vi "Volt Reader Trigger9.vi"() -> ()   [LabVIEW 2014]
uses:
  Enum State Machine Typedef.ctl
  <vilib>/Utility/error.llb/DialogType.ctl
  <vilib>/_DAQmxBase/Internals/DAQmxBase Create Channel (AI-Voltage-Basic).vi
  <vilib>/_DAQmxBase/Internals/DAQmxBase Timing (Sample Clock).vi
  <vilib>/measure/mamon.llb/Trigger Detection for 1 Channel.vi
  <vilib>/_DAQmxBase/Internals/DAQmxBase Read (Analog 2D DBL NChan NSamp).vi
  <vilib>/measure/NI_MAPro.lvlib
panel:
  out "trigger location":dbl
  in  "Timeout (in iterations)":i16
  out "State":T1
  out "Raw Waveform":waveform(dbl)(graph)
  out "Waveform Graph":waveform(dbl)(graph)
  in  "Buffer (Seconds)":dbl
  out "Threshold":dbl
  in  "units":i32(ring)=10348 items=["Volts"=10348, "From Custom Scale"=10065]
  in  "stop":bool
  in  "physical channels":tag
  in  "maximum value":dbl=5.0 format="%0.2f"
  in  "minimum value":dbl=-5.0 format="%0.2f"
  in  "rate":i32=1000 caption="Sample Rate"
  # "The inputs above MUST BE\nPreset before running"
  # "NOTE: Just change the Y axis value"
  # "Make Sure that Buffer does not equal 0"
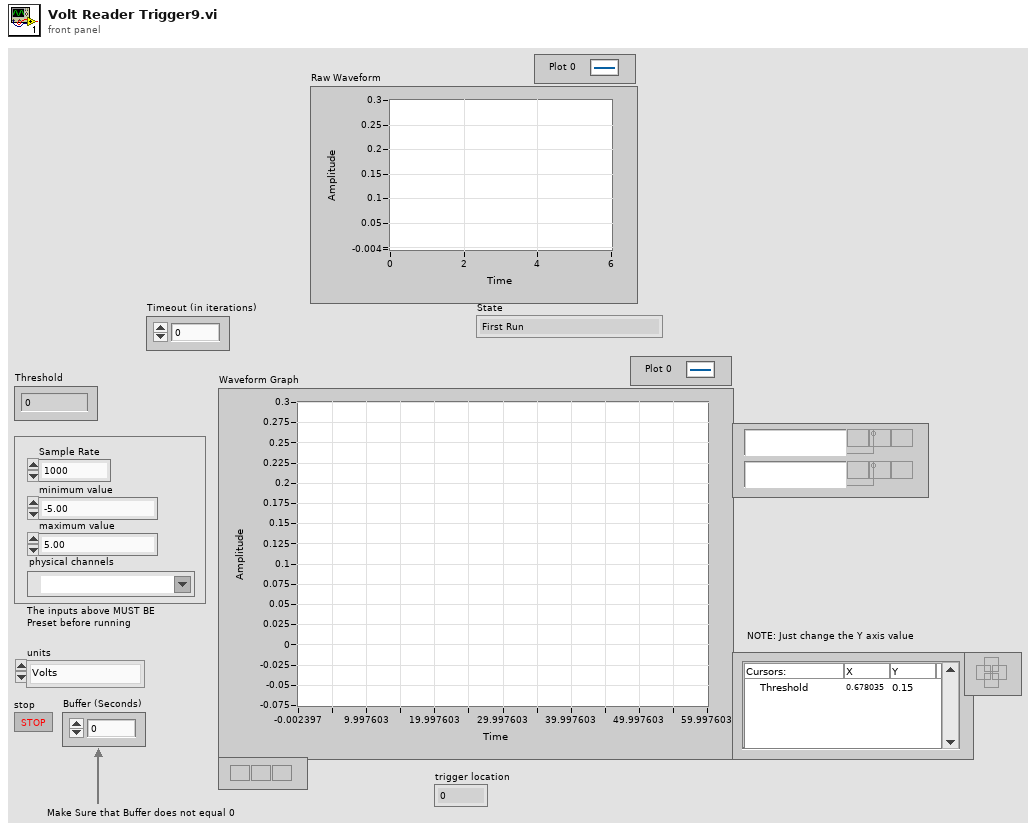
[diagram p1: front panel]
types:
  T1 = typedef "Enum State Machine Typedef.ctl" = enum16{"First Run", "Gather and Edit Data", "Find Max with Gather Data", "Trigger Occured", "Found the Max", "Just Displayed", "The Max is in the Middle", "Base State", "Timeout"}
  T2 = typedef "DialogType.ctl" = u16
  T3 = typedef "LVCursorListTypeDef.ctl" = cluster{"Name":string, "Color":u32, "Style":u8, "Point Style":u8, "Name Visible":bool, "Allow Drag":bool, "Cursor Mode":u32, "Plot":i32, "Index":i32, "Position":cluster{"X":dbl, "Y":dbl}, "X Scale":u32, "Y Scale":u32, "Watch Plots":i32[], "Watch All Plots":bool, "Plot Area":i32, "Label Offset":cluster{"X":dbl, "Y":dbl}}[]
  T4 = cluster{"Name":string, "Color":u32, "Style":u8, "Point Style":u8, "Name Visible":bool, "Allow Drag":bool, "Cursor Mode":u32, "Plot":i32, "Index":i32, "Position":cluster{"X":dbl, "Y":dbl}, "X Scale":u32, "Y Scale":u32, "Watch Plots":i32[], "Watch All Plots":bool, "Plot Area":i32, "Label Offset":cluster{"X":dbl, "Y":dbl}}
  T5 = enum16{"In the Center Range", "Before the Center Range", "After the Center Range"}
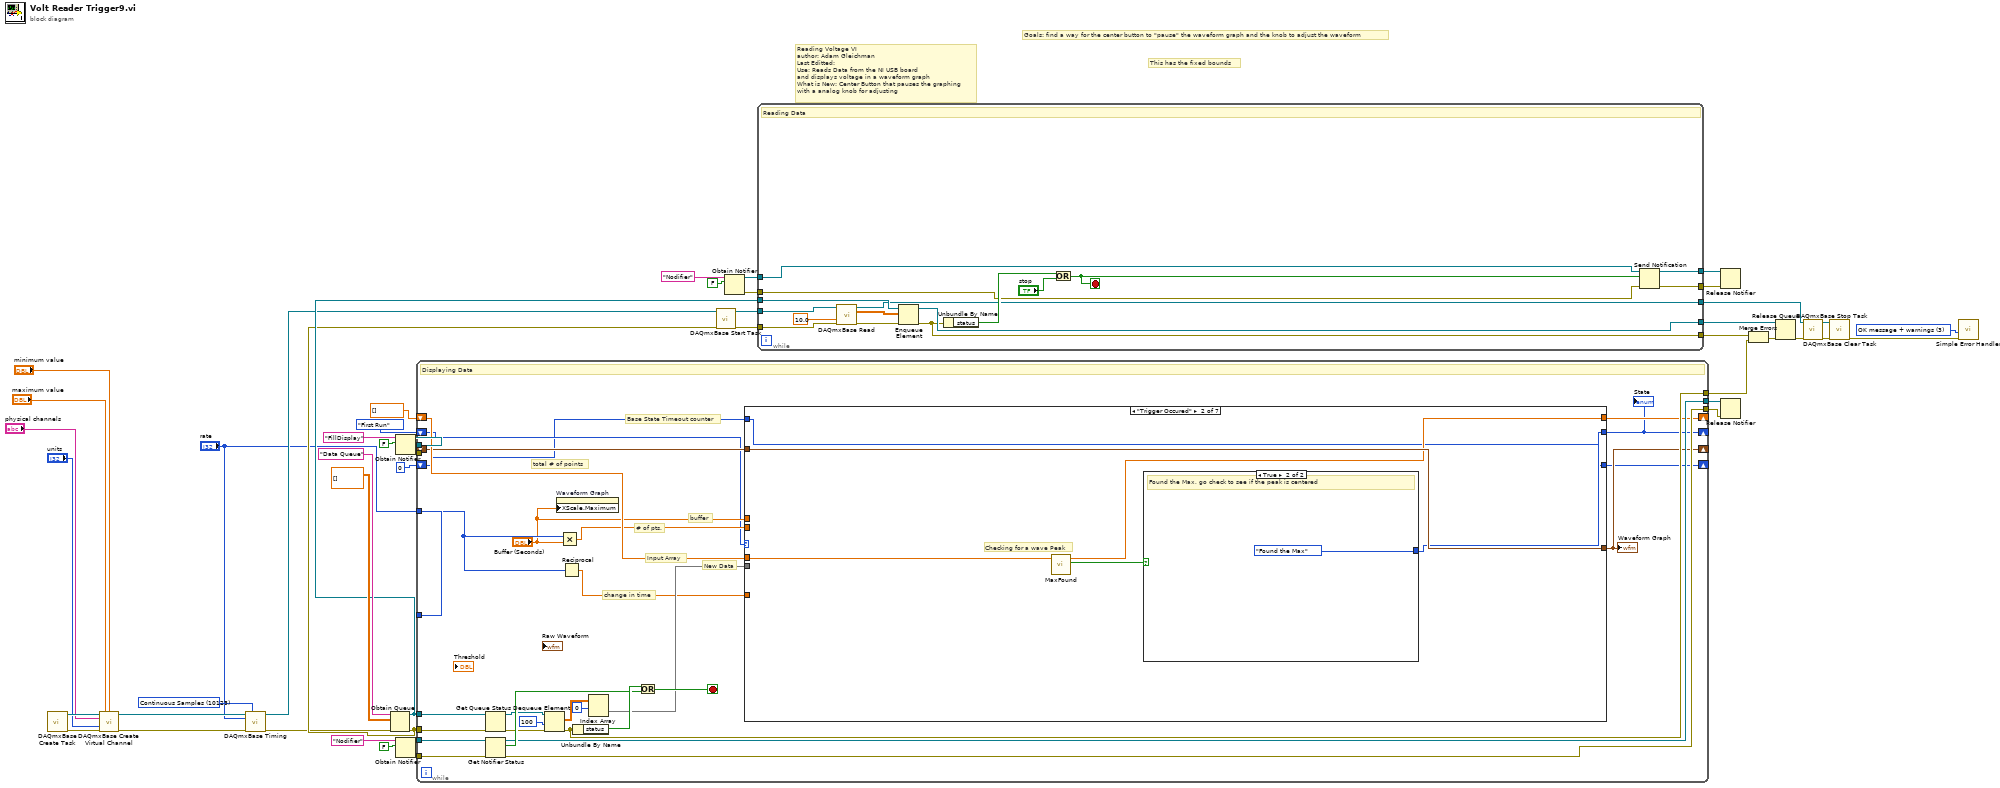
[diagram p0: block diagram]
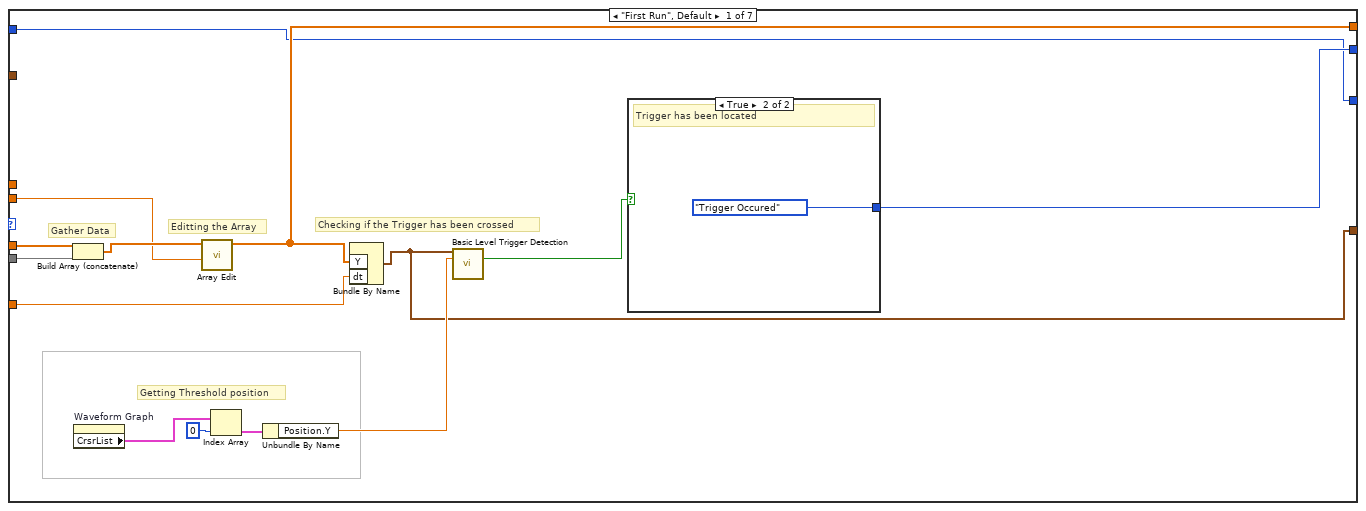
[diagram p2: hidden frame]
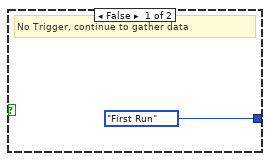
[diagram p3: hidden frame]
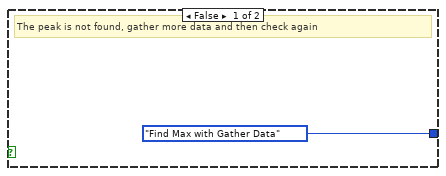
[diagram p4: hidden frame]
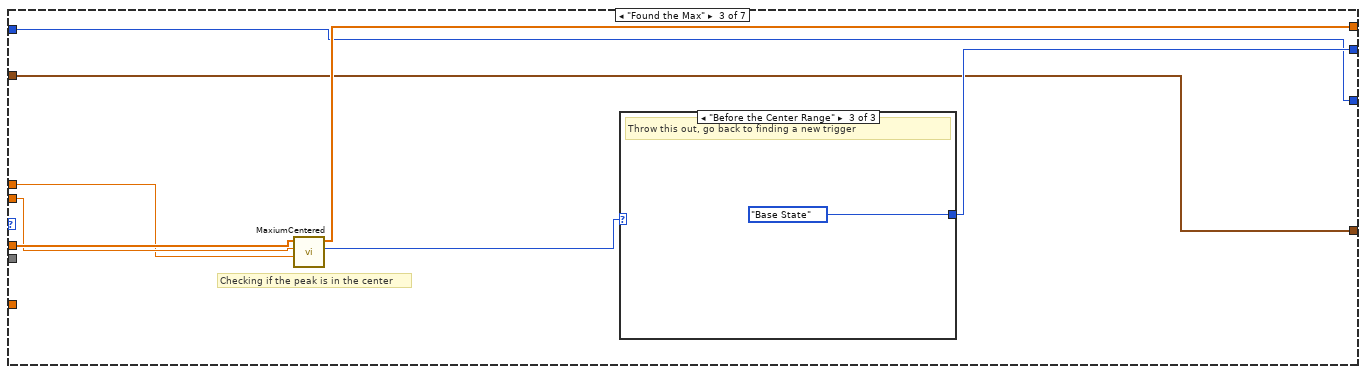
[diagram p5: hidden frame]
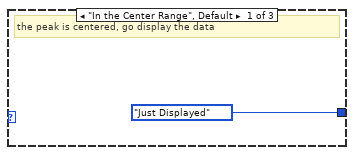
[diagram p6: hidden frame]
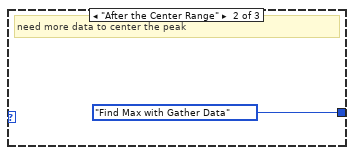
[diagram p7: hidden frame]
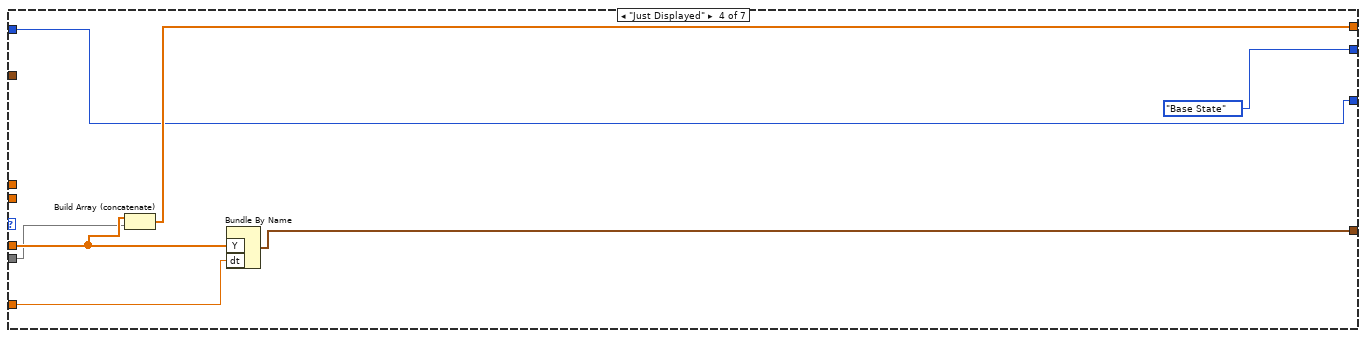
[diagram p8: hidden frame]
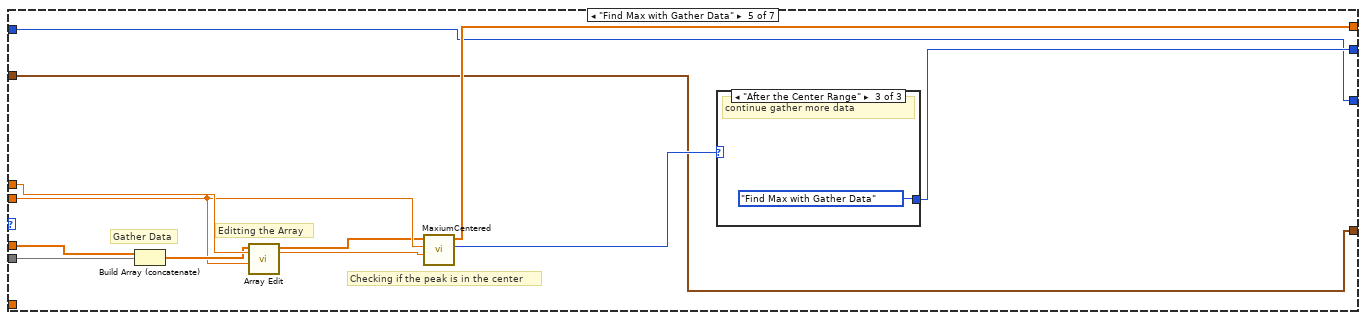
[diagram p9: hidden frame]
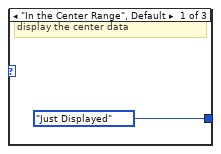
[diagram p10: hidden frame]
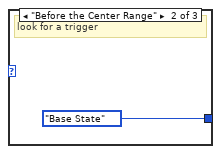
[diagram p11: hidden frame]
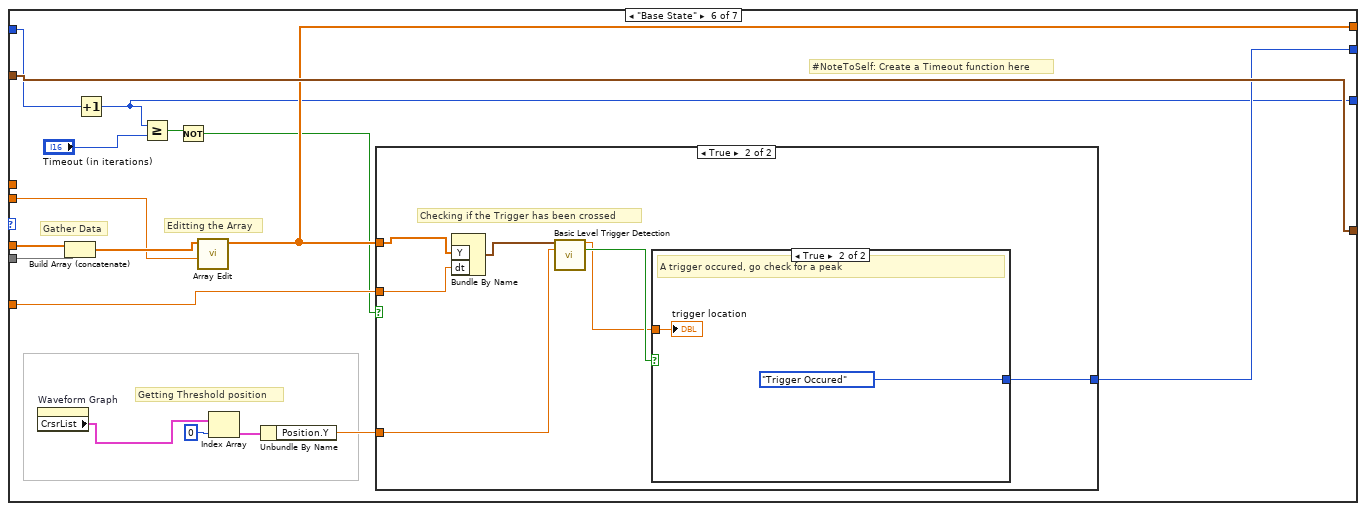
[diagram p12: hidden frame]
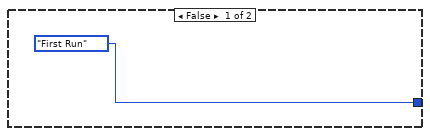
[diagram p13: hidden frame]
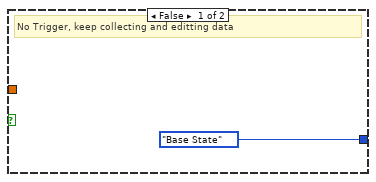
[diagram p14: hidden frame]
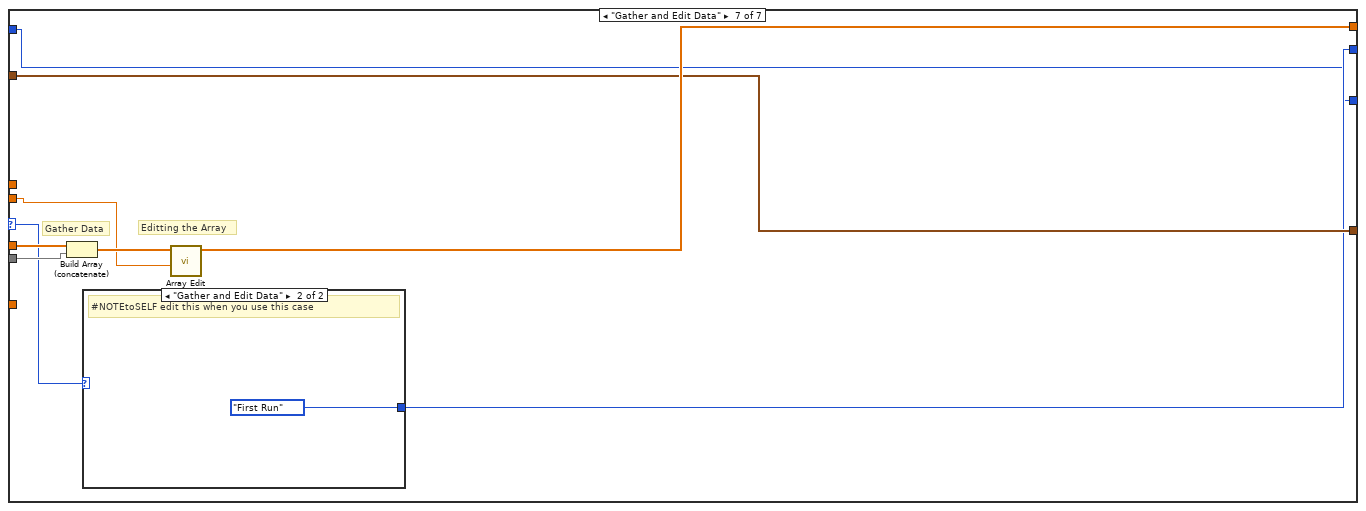
[diagram p15: hidden frame]
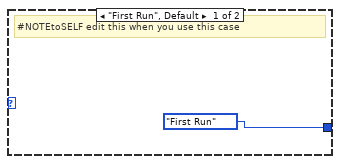
[diagram p16: hidden frame]
diagram:
  w24 = 10123 items=["Finite Samples"=10178, "Continuous Samples"=10123, "Hardware Timed Single Point"=12522] ("sample mode")
  w26 = T2 3 items=["no dialog", "OK message", "continue or stop message", "OK message + warnings", "continue/stop + warnings"] ("type of dialog (OK msg:1)")
  # "Goals: find a way for the center button to \"pause\" the waveform graph and the knob to adjust the waveform"
  # "This has the fixed bounds"
  # "Reading Voltage VI\nauthor: Adam Gleichman\nLast Editted: \nUse: Reads Data from the NI USB board\nand displays voltage in a waveform graph\nWhat is New: Center Button that pauses the graphing\nwith a analog knob for adjusting"
  n1 = call <vilib>:"DAQmxBase Create Task.vi"() -> ("task out"=w46:refnum<k21>, "error out"=w45:errorcluster)  [unwired: 5 in, 9 out]
  n2 = call-poly <vilib>:"DAQmxBase Create Virtual Channel.vi"("task in"=w46, "maximum value"="maximum value", "minimum value"="minimum value", "physical channels"="physical channels", "units"="units", "error in"=w45) -> ("task out"=w43:refnum<k21>, "error out"=w44:errorcluster)  [unwired: 3 in, 5 out]
  n3 = call-poly <vilib>:"DAQmxBase Timing.vi"("task/channels in"=w43, "sample mode"=w24, "rate"="rate", "error in"=w44) -> ("task out"=w12:refnum<k21>, "error out"=w11:errorcluster)  [unwired: 3 in, 7 out]
  n4 = Obtain Queue(name (unnamed)="Data Queue", element data type=dbl[][] [] ("data"), error in (no error)=w11) -> (queue out=w33:refnum<queue>, error out=w32:errorcluster)  [unwired: 2 in, 1 out]
  n5 = Obtain Notifier(name (unnamed)="FillDisplay", notification data type=FALSE) -> (notifier out=w8:refnum<notifier>, error out=w7:errorcluster)  [unwired: 2 in, 1 out]
  n6 = Obtain Notifier(name (unnamed)="Nodifier", notification data type=FALSE) -> (notifier out=w17:refnum<notifier>, error out=w15:errorcluster)  [unwired: 2 in, 1 out]
  n7 = while {
    tunnel: w33 -> [w75]
    tunnel: w32 -> [w64]
    tunnel: [w73] -> w31
    tunnel: w17 -> [w70]
    tunnel: w15 -> [w69]
    tunnel: [w67] -> w13
    tunnel: [w66] -> w14
    tunnel: "rate" -> [_]
    tunnel: "rate" -> [w60]
    shift-right: [w51] -> _
    shift-left: dbl[] [] -> [w59]
    tunnel: w8 -> [_]
    tunnel: w7 -> [_]
    shift-right: [w50] -> _
    shift-left: Enum_State_Machine_Typedef."First Run" -> [w53]
    shift-right: [w52] -> _
    shift-left: _ -> [w55]
    shift-right: [w48] -> _
    shift-left: 0 -> [w49]
    stop <- w71 stop-if-true
    # "Base State Timeout counter"
    # "change in time"
    # "buffer"
    # "New Data"
    # "Input Array"
    # "# of pts."
    # "total # of points"
    # "Displaying Data"
    n8 = Get Queue Status(queue=w75, error in (no error)=w64) -> (queue out=w65:refnum<queue>, error out=w63:errorcluster)  [unwired: 1 in, 6 out]
    n9 = Get Notifier Status(notifier=w70, error in (no error)=w69) -> (notifier out=w67:refnum<notifier>, current notification=w68:bool, error out=w66:errorcluster)  [unwired: 2 out]
    n10 = Dequeue Element(queue=w65, timeout in ms (-1)=100, error in (no error)=w63) -> (element=w61:dbl[][], error out=w73:errorcluster)  [unwired: 2 out]
    n11 = property on="Waveform Graph" class="WFGraph (strict)"("XScale.Maximum"="Buffer (Seconds)") -> ()  [unwired: 2 in, 2 out]
    n12 = Multiply(x=w60, y="Buffer (Seconds)") -> (x*y=w56:dbl)
    n13 = Reciprocal(x=w60) -> (1/x=w57:dbl)
    n14 = Unbundle By Name(w73) -> ("status"=w72:bool)
    n15 = Index Array(array=w61, index (row)=0 ("index")) -> (element=w58:dbl[])  [unwired: 1 in]
    n16 = Or(x=w72, y=w68) -> (x .or. y?=w71:bool)
    n17 = case shown="\"Trigger Occured\"" w53 {
      selector: w53 -> [_ _ _ _ _ _ w164]
      tunnel: w59 -> [w89 w97 w107 w116 w128 w148 w168]
      tunnel: w58 -> [w88 _ _ w115 w127 w147 w167]
      tunnel: w57 -> [w82 _ _ w117 _ w141 _]
      tunnel: w56 -> [w86 _ w106 _ w124 w145 w165]
      tunnel: [w79 w96 w101 w113 w119 w140 w162] -> w52
      tunnel: w55 -> [_ w96 w101 _ w119 w140 w162]
      tunnel: "Buffer (Seconds)" -> [_ _ w105 _ w126 _ _]
      tunnel: [w78 w94 w104 w114 w121 w138 w163] -> w51
      tunnel: [w77 w93 w102 Enum_State_Machine_Typedef."Base State" w120 w139 w161] -> w50
      tunnel: w49 -> [w76 w92 w100 w111 w118 w136 w160]
      tunnel: [w76 w92 w100 w111 w118 w132 w160] -> w48
      frame "First Run", Default {
        # "Checking if the Trigger has been crossed"
        # "Getting Threshold position"
        # "Editting the Array"
        # "Gather Data"
        n18 = Build Array (concatenate)(w89, w88) -> (w87:dbl[])
        n19 = property on="Waveform Graph" class="WFGraph (strict)"() -> ("CrsrList"=w84:T3)  [unwired: 2 in, 2 out]
        n20 = call "Array Edit.vi"("Number of Points"=w86, "Y-values"=w87) -> ("Editted Y Values"=w78:dbl[])  [unwired: 9 in]
        n21 = Index Array(array=w84, index=0) -> (element=w85:T4)
        n22 = Unbundle By Name(w85) -> ("Position.Y"=w81:dbl)
        n23 = Bundle By Name("Y"=w78, "dt"=w82) -> (w79:waveform(dbl))  [unwired: 1 in]
        n24 = call-poly <vilib>:"Basic Level Trigger Detection.vi"("signal in"=w79, "level"=w81) -> ("trigger detected?"=w80:bool)  [unwired: 11 in, 2 out]
        n25 = case shown="True" w80 {
          tunnel: [Enum_State_Machine_Typedef."First Run" Enum_State_Machine_Typedef."Trigger Occured"] -> w77
          frame False {
            # "No Trigger, continue to gather data"
          }
          frame True {
            # "Trigger has been located"
          }
        }
      }
      frame "Trigger Occured" {
        # "Checking for a wave Peak"
        n26 = call "MaxFound.vi"("Input Y Values"=w97) -> ("Max?"=w95:bool, "Output Y Values"=w94:dbl[])  [unwired: 9 in]
        n27 = case shown="True" w95 {
          tunnel: [Enum_State_Machine_Typedef."Find Max with Gather Data" Enum_State_Machine_Typedef."Found the Max"] -> w93
          frame False {
            # "The peak is not found, gather more data and then check again"
          }
          frame True {
            # "Found the Max, go check to see if the peak is centered"
          }
        }
      }
      frame "Found the Max" {
        # "Checking if the peak is in the center"
        n28 = call "MaxiumCentered.vi"("Buffer"=w105, "Number of Points"=w106, "Input Y Values"=w107) -> ("State output"=w103:T5, "Output Y Values"=w104:dbl[])  [unwired: 7 in]
        n29 = case shown="\"Before the Center Range\"" w103 {
          tunnel: [Enum_State_Machine_Typedef."Just Displayed" Enum_State_Machine_Typedef."Find Max with Gather Data" Enum_State_Machine_Typedef."Base State"] -> w102
          frame "In the Center Range", Default {
            # "the peak is centered, go display the data"
          }
          frame "After the Center Range" {
            # "need more data to center the peak"
          }
          frame "Before the Center Range" {
            # "Throw this out, go back to finding a new trigger"
          }
        }
      }
      frame "Just Displayed" {
        n30 = Build Array (concatenate)(w116, w115) -> (w114:dbl[])
        n31 = Bundle By Name("Y"=w116, "dt"=w117) -> (w113:waveform(dbl))  [unwired: 1 in]
      }
      frame "Find Max with Gather Data" {
        # "Editting the Array"
        # "Gather Data"
        # "Checking if the peak is in the center"
        n32 = Build Array (concatenate)(w128, w127) -> (w125:dbl[])
        n33 = call "Array Edit.vi"("Number of Points"=w124, "Y-values"=w125) -> ("Editted Y Values"=w123:dbl[])  [unwired: 9 in]
        n34 = call "MaxiumCentered.vi"("Buffer"=w126, "Number of Points"=w124, "Input Y Values"=w123) -> ("State output"=w122:T5, "Output Y Values"=w121:dbl[])  [unwired: 7 in]
        n35 = case shown="\"After the Center Range\"" w122 {
          tunnel: [Enum_State_Machine_Typedef."Just Displayed" Enum_State_Machine_Typedef."Base State" Enum_State_Machine_Typedef."Find Max with Gather Data"] -> w120
          frame "In the Center Range", Default {
            # "display the center data"
          }
          frame "Before the Center Range" {
            # "look for a trigger"
          }
          frame "After the Center Range" {
            # "continue gather more data"
          }
        }
      }
      frame "Base State" {
        # "#NoteToSelf: Create a Timeout function here"
        # "Getting Threshold position"
        # "Editting the Array"
        # "Gather Data"
        n36 = property on="Waveform Graph" class="WFGraph (strict)"() -> ("CrsrList"=w137:T3)  [unwired: 2 in, 2 out]
        n37 = Build Array (concatenate)(w148, w147) -> (w146:dbl[])
        n38 = Increment(x=w136) -> (x+1=w132:i32)
        n39 = Greater Or Equal?(x=w132, y="Timeout (in iterations)") -> (x >= y?=w134:bool)
        n40 = Not(x=w134) -> (.not. x?=w133:bool)
        n41 = call "Array Edit.vi"("Number of Points"=w145, "Y-values"=w146) -> ("Editted Y Values"=w138:dbl[])  [unwired: 9 in]
        n42 = Index Array(array=w137, index=0) -> (element=w144:T4)
        n43 = Unbundle By Name(w144) -> ("Position.Y"=w142:dbl)
        n44 = case shown="True" w133 {
          tunnel: w142 -> [_ w155]
          tunnel: w141 -> [_ w154]
          tunnel: [Enum_State_Machine_Typedef."First Run" w152] -> w139
          tunnel: w138 -> [_ w151]
          frame False {
          }
          frame True {
            # "Checking if the Trigger has been crossed"
            n45 = Bundle By Name("Y"=w151, "dt"=w154) -> (w156:waveform(dbl))  [unwired: 1 in]
            n46 = call-poly <vilib>:"Basic Level Trigger Detection.vi"("signal in"=w156, "level"=w155) -> ("trigger location"=w150:dbl, "trigger detected?"=w153:bool)  [unwired: 11 in, 1 out]
            n47 = case shown="True" w153 {
              tunnel: [Enum_State_Machine_Typedef."Base State" Enum_State_Machine_Typedef."Trigger Occured"] -> w152
              tunnel: w150 -> [_ w158]
              frame False {
                # "No Trigger, keep collecting and editting data"
              }
              frame True {
                # "A trigger occured, go check for a peak"
                "trigger location" <- w158
              }
            }
          }
        }
      }
      frame "Gather and Edit Data" {
        # "Editting the Array"
        # "Gather Data"
        n48 = Build Array (concatenate)(w168, w167) -> (w166:dbl[])
        n49 = case shown="\"Gather and Edit Data\"" w164 {
          tunnel: [Enum_State_Machine_Typedef."First Run" Enum_State_Machine_Typedef."First Run"] -> w161
          frame "First Run", Default {
            # "#NOTEtoSELF edit this when you use this case"
          }
          frame "Gather and Edit Data" {
            # "#NOTEtoSELF edit this when you use this case"
          }
        }
        n50 = call "Array Edit.vi"("Number of Points"=w165, "Y-values"=w166) -> ("Editted Y Values"=w163:dbl[])  [unwired: 9 in]
      }
    }
    "Waveform Graph" <- w52
    "State" <- w50
  }
  n51 = call <vilib>:"DAQmxBase Start Task.vi"("task/channels in"=w12, "error in"=w32) -> ("task out"=w41:refnum<k21>, "error out"=w42:errorcluster)  [unwired: 12 out]
  n52 = Obtain Notifier(name (unnamed)="Nodifier", notification data type=FALSE) -> (notifier out=w20:refnum<notifier>, error out=w19:errorcluster)  [unwired: 2 in, 1 out]
  n53 = while "Data Reading Loop" {
    tunnel: w42 -> [w185]
    tunnel: w41 -> [w186]
    tunnel: w33 -> [w183]
    tunnel: [w180] -> w36
    tunnel: [w178] -> w35
    tunnel: [w176] -> w23
    tunnel: w20 -> [w174]
    tunnel: w19 -> [w173]
    tunnel: [w172] -> w10
    tunnel: [w171] -> w9
    stop <- w175 stop-if-true
    # "Reading Data"
    n54 = call-poly <vilib>:"DAQmxBase Read.vi"("task/channels in"=w186, "timeout"=10.0, "error in"=w185) -> ("task out"=w176:refnum<k21>, "data"=w181:dbl[][], "error out"=w184:errorcluster)  [unwired: 10 in]
    n55 = Enqueue Element(queue=w183, element=w181, error in (no error)=w184) -> (queue out=w180:refnum<queue>, error out=w178:errorcluster)  [unwired: 1 in, 1 out]
    n56 = Unbundle By Name(w178) -> ("status"=w177:bool)
    n57 = Or(x=w177, y="stop") -> (x .or. y?=w175:bool)
    n58 = Send Notification(notification=w175, notifier=w174, error in (no error)=w173) -> (notifier out=w172:refnum<notifier>, error out=w171:errorcluster)
  }
  n59 = Release Notifier(notifier=w10, error in (no error)=w9) -> ()  [unwired: 1 in, 3 out]
  n60 = Release Notifier(notifier=w13, error in (no error)=w14) -> ()  [unwired: 1 in, 3 out]
  n61 = Merge Errors(w35, w31) -> (w34:errorcluster)
  n62 = Release Queue(queue=w36, error in (no error)=w34) -> (error out=w30:errorcluster)  [unwired: 1 in, 2 out]
  n63 = call <vilib>:"DAQmxBase Stop Task.vi"("task/channels in"=w23, "error in"=w30) -> ("task out"=w29:refnum<k21>, "error out"=w28:errorcluster)  [unwired: 12 in]
  n64 = call <vilib>:"DAQmxBase Clear Task.vi"("task in"=w29, "error in"=w28) -> ("error out"=w27:errorcluster)  [unwired: 13 in]
  n65 = call <vilib>:"Simple Error Handler.vi"("type of dialog (OK msg:1)"=w26, "error in (no error)"=w27) -> ()  [unwired: 3 in, 5 out]
